vi "wcs_rotate_reverse.vi"(8 "theta":dbl, 9 "phi":dbl, 11 "Astrometry":T1) -> (0 "lat":dbl, 1 "lon":dbl)   [LabVIEW 2019]
panel:
  out "b2":dbl
  out "b0":dbl
  out "b1":dbl
  out "theta1":dbl
  out "phi1":dbl
  out "n":dbl
  out "m":dbl
  out "l":dbl
  out "rr":dbl[][](array[numeric])
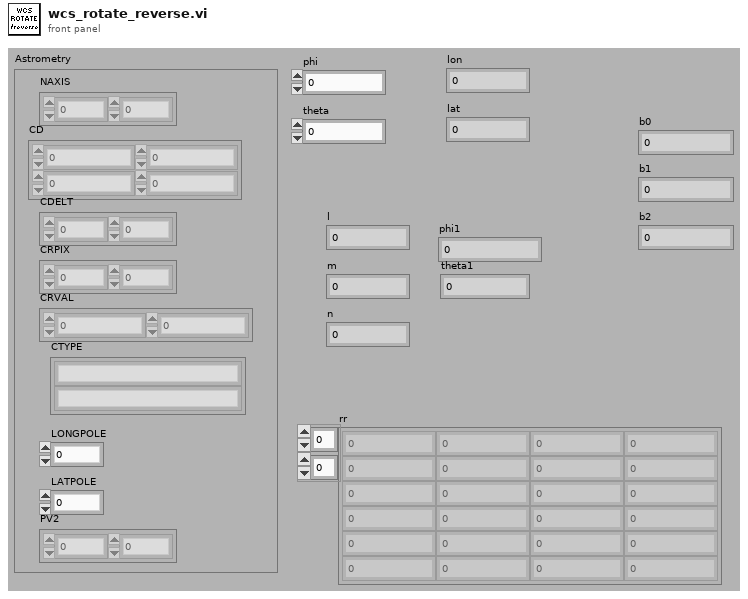
[diagram p1: front panel]
types:
  T1 = cluster{"NAXIS":dbl[], "CD":dbl[][], "CDELT":dbl[], "CRPIX":dbl[], "CTYPE":string[], "CRVAL":dbl[], "LONGPOLE":dbl, "LATPOLE":dbl, "PV2":dbl[]}
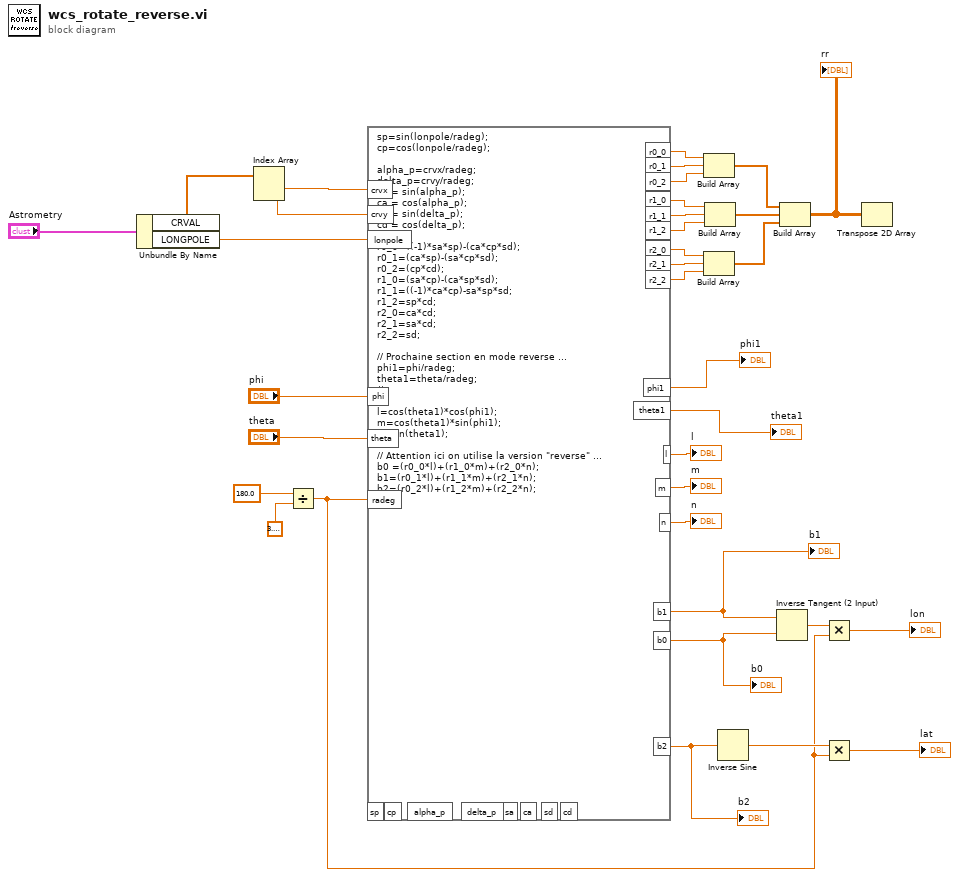
[diagram p0: block diagram]
diagram:
  n1 = Unbundle By Name("Astrometry") -> ("CRVAL"=w33:dbl[], "LONGPOLE"=w34:dbl)
  n2 = Index Array(array=w33) -> (element #1=w32:dbl, element #2=w31:dbl)  [unwired: 2 in]
  n3 = Divide(x=180.0, y=3.141592653589793) -> (x/y=w6:dbl)
  n4 = formula code="sp=sin(lonpole/radeg);\ncp=cos(lonpole/radeg);\n\nalpha_p=crvx/radeg;\ndelta_p=crvy/radeg;\nsa = sin(alpha_p);\nca = cos(alpha_p);\nsd = sin(delta_p);\ncd = cos(delta_p);\n\nr0_0=((-1)*sa*sp)-(ca*cp*sd);\nr0_1=(ca*sp)-(sa*cp*sd);\nr0_2=(cp*cd);\nr1_0=(sa*cp)-(ca*sp*sd);\nr1_1=((-1)*ca*cp)-sa*sp*sd;\nr1_2=sp*cd;\nr2_0=ca*cd;\nr2_1=sa*cd;\nr2_2=sd;\n\n// Prochaine section en mode reverse ...\nphi1=phi/radeg;\ntheta1=theta/radeg;\n//\n\nl=cos(theta1)*cos(phi1);\nm=cos(theta1)*sin(phi1);\nn=sin(theta1);\n\n// Attention ici on utilise la version \"reverse\" ...\nb0 =(r0_0*l)+(r1_0*m)+(r2_0*n);\nb1=(r0_1*l)+(r1_1*m)+(r2_1*n);\nb2=(r0_2*l)+(r1_2*m)+(r2_2*n);\n//"("lonpole"=w34, "crvx"=w32, "crvy"=w31, "radeg"=w6, "phi"="phi", "theta"="theta") -> ("r0_0"=w30:dbl, "r0_1"=w29:dbl, "r0_2"=w28:dbl, "r1_0"=w27:dbl, "r1_1"=w26:dbl, "r1_2"=w25:dbl, "r2_0"=w24:dbl, "r2_1"=w23:dbl, "r2_2"=w22:dbl, "phi1"=→"phi1":dbl, "theta1"=→"theta1":dbl, "l"=→"l":dbl, "m"=→"m":dbl, "n"=→"n":dbl, "b0"=w2:dbl, "b1"=w8:dbl, "b2"=w1:dbl)  [unwired: 8 out]
  "b1" <- w8
  "b0" <- w2
  "b2" <- w1
  n5 = Build Array(w30, w29, w28) -> (w21:dbl[])
  n6 = Build Array(w24, w23, w22) -> (w19:dbl[])
  n7 = Build Array(w27, w26, w25) -> (w20:dbl[])
  n8 = Inverse Sine(1:w1) -> (0:w10:dbl)
  n9 = Inverse Tangent (2 Input)(1:w2, 2:w8) -> (0:w7:dbl)
  n10 = Build Array(w21, w20, w19) -> (w16:dbl[][])
  "rr" <- w16
  n11 = Multiply(x=w7, y=w6) -> (x*y=→"lon":dbl)
  n12 = Multiply(x=w10, y=w6) -> (x*y=→"lat":dbl)
  n13 = Transpose 2D Array(2D array=w16) -> ()  [unwired: 1 out]
